vi "OE2052_Configure Channel Out.vi"(7 "OE2052_Configure Channel Out":T1={"Channel Output"=0, "Channel Source"=0, "Offset(%)"=0.0, "Expand"=1, "AUX OUT"=1.0, "Sensitivity "=24} {"Sensitivity" items=["1 nV/fA", "2 nV/fA", "5 nV/fA", "10 nV/fA", "20 nV/fA", "50 nV/fA", "100 nV/fA", "200 nV/fA", "500 nV/fA", "1 uV/pA", "2 uV/pA", "5 uV/pA", "10 uV/pA", "20 uV/pA", "50 uV/pA", "100 uV/pA", "200 uV/pA", "500 uV/pA", "1 mV/nA", "2 mV/nA", "5 mV/nA", "10 mV/nA", "20 mV/nA", "50 mV/nA", "100 mV/nA", "200 mV/nA", "500 mV/nA", "1 V/uA"]; "AUX OUT" min=-10.0 max=10.0 format="%#.3g"; "Expand" min=1 max=10000; "Offset(%)" min=-100.0 max=100.0 format="%#_5g"; "Channel Source" items=["AUXOUT", "X1", "Y1", "R1", "θ1", "X2", "Y2", "R2", "θ2", "Frequency1", "Frequency2", "AUX-IN1", "AUX-IN2", "AUX-IN3", "AUX-IN4", "X3", "Y3", "R3", "Xita3", "X4", "Y4", "R4", "Xita4"]; "Channel Output" items=["CH1", "CH2", "CH3", "CH4"]}, 8 "Error in (no error)":errorcluster caption="error out（no error）", 9 "Remote Mode":u16(ring) items=["USB"=0, "RS232"=1, "Ethernet"=3], 10 "Connection ID in":refnum<k5>, 11 "VISA resource name":refnum<visa-resource-name>) -> (0 "Error out":errorcluster caption="error out", 1 "Output String":string, 2 "Connection ID out":refnum<k5>, 3 "VISA resource  out":refnum<visa-resource-name>)   [LabVIEW 2011]
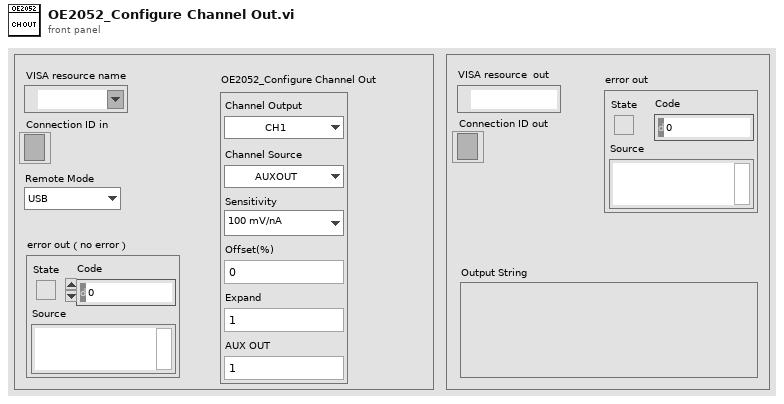
[diagram p1: front panel]
types:
  T1 = cluster{"Channel Output":u16, "Channel Source":u16, "Offset(%)":dbl, "Expand":u16, "AUX OUT":dbl, "Sensitivity ":u16}
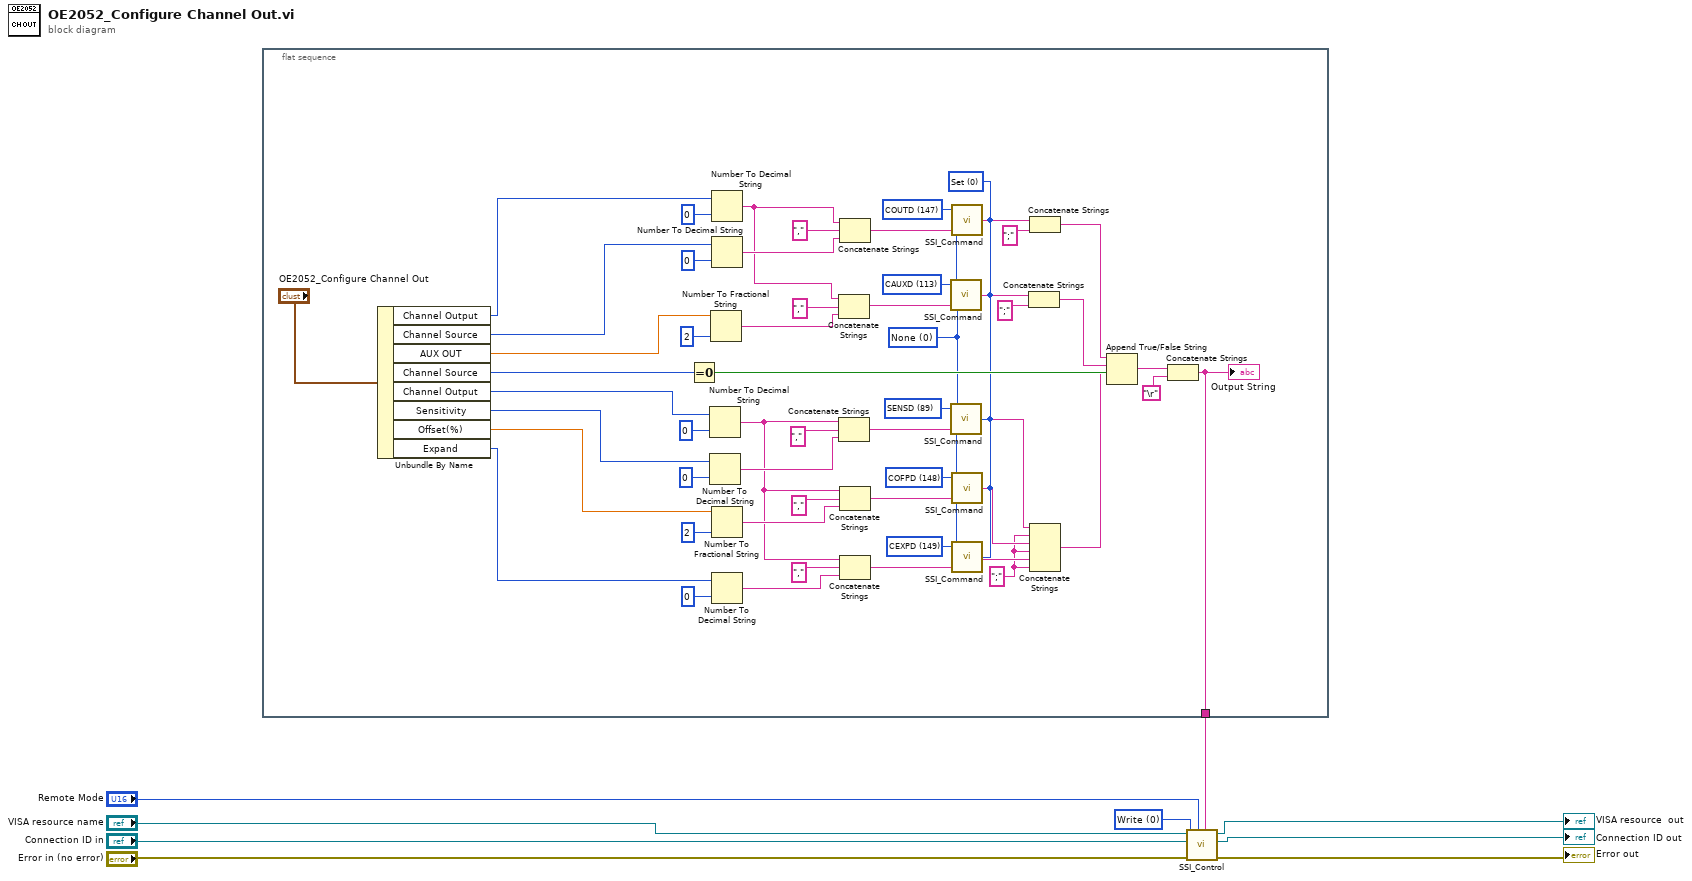
[diagram p0: block diagram]
diagram:
  w2 = u16 0 items=["Write", "Read"] ("Control")
  n1 = flat-sequence {
    tunnel: [w40] -> w1
    frame #0 {
      w11 = u16 0 items=["A"=1, "B"=2, "None"=0] ("channel")
      w20 = u16 149 items=["ISRC", "IGND", "ICPL", "ILIN", "PHAS", "FMOD", "RSLP", "FREQ", "SWPT", "SLLM", "SULM", "SSLL", "SSLG", "STLM", "SWRM", "IRNG", "SENS", "RMOD", "OFLT", "OFSL", "SYNC", "DMOD", "HARM", "DARB", "SWVT", "SLVL", "SVLL", "SVUL", "SVSL", "SVSG", "SVTM", "SVRM", "RALL", "SNAP", "OUTP", "OAUX", "COUT", "CAUX", "COFP", "CEXP", "FPOP", "OEXP", "*IDN", "*RST", "OVLD", "INOV", "GNOV", "*PLL", "SSET", "RSET", "AGAN", "APHS", "ARSV", "ASCL", "EQCD", "EQCS", "SPED", "SRAT", "SLEN", "SSLE", "STRG", "SPRM", "STRD", "PAUS", "REST", "SPTS", "TRCA", "TEMP", "RSTU", "INHZ", "DEQU", "SADD", "ARNG", "CSPE", "ISRCD", "IGNDD", "ICPLD", "ILIND", "PHASD", "FMODD", "RSLPD", "FREQD", "SWPTD", "SLLMD", "SULMD", "SSLLD", "SSLGD", "STLMD", "SWRMD", "SENSD", "RMODD", "OFLTD", "OFSLD", "SYNCD", "HARMD", "EQCDD", "EQCSD", "SNAPD", "OUTPD", "SWVTD", "SLVLD", "SVLLD", "SVULD", "SVSLD", "SVSGD", "SVTMD", "SVRMD", "SVDCD", "ARSVD", "AGAND", "APHSD", "ASCLD", "FPOPD", "CAUXD", "OEXPD", "SPEDD", "SRATD", "SLEND", "SSLED", "STRGD", "SPRMD", "STRDD", "PAUSD", "RESTD", "SPTSD", "TRCAD", "*IDND", "*RSTD", "INOVD", "GNOVD", "*PLLD", "SSETD", "RSETD", "RALLD", "NIPA", "NSMA", "NGWA", "NMAC", "NMOD", "TRIG", "TRCB", "INHZD", "ISAMD", "IRAGD", "RRAGD", "SOFFD", "DMODD", "COUTD", "COFPD", "CEXPD", "ARNGD", "OAUXD", "TRIM", "SUITD", "SNHZD", "AOFSD"] ("Command Type")
      w21 = u16 148 items=["ISRC", "IGND", "ICPL", "ILIN", "PHAS", "FMOD", "RSLP", "FREQ", "SWPT", "SLLM", "SULM", "SSLL", "SSLG", "STLM", "SWRM", "IRNG", "SENS", "RMOD", "OFLT", "OFSL", "SYNC", "DMOD", "HARM", "DARB", "SWVT", "SLVL", "SVLL", "SVUL", "SVSL", "SVSG", "SVTM", "SVRM", "RALL", "SNAP", "OUTP", "OAUX", "COUT", "CAUX", "COFP", "CEXP", "FPOP", "OEXP", "*IDN", "*RST", "OVLD", "INOV", "GNOV", "*PLL", "SSET", "RSET", "AGAN", "APHS", "ARSV", "ASCL", "EQCD", "EQCS", "SPED", "SRAT", "SLEN", "SSLE", "STRG", "SPRM", "STRD", "PAUS", "REST", "SPTS", "TRCA", "TEMP", "RSTU", "INHZ", "DEQU", "SADD", "ARNG", "CSPE", "ISRCD", "IGNDD", "ICPLD", "ILIND", "PHASD", "FMODD", "RSLPD", "FREQD", "SWPTD", "SLLMD", "SULMD", "SSLLD", "SSLGD", "STLMD", "SWRMD", "SENSD", "RMODD", "OFLTD", "OFSLD", "SYNCD", "HARMD", "EQCDD", "EQCSD", "SNAPD", "OUTPD", "SWVTD", "SLVLD", "SVLLD", "SVULD", "SVSLD", "SVSGD", "SVTMD", "SVRMD", "SVDCD", "ARSVD", "AGAND", "APHSD", "ASCLD", "FPOPD", "CAUXD", "OEXPD", "SPEDD", "SRATD", "SLEND", "SSLED", "STRGD", "SPRMD", "STRDD", "PAUSD", "RESTD", "SPTSD", "TRCAD", "*IDND", "*RSTD", "INOVD", "GNOVD", "*PLLD", "SSETD", "RSETD", "RALLD", "NIPA", "NSMA", "NGWA", "NMAC", "NMOD", "TRIG", "TRCB", "INHZD", "ISAMD", "IRAGD", "RRAGD", "SOFFD", "DMODD", "COUTD", "COFPD", "CEXPD", "ARNGD", "OAUXD", "TRIM", "SUITD", "SNHZD", "AOFSD"] ("Command Type")
      w22 = u16 89 items=["ISRC", "IGND", "ICPL", "ILIN", "PHAS", "FMOD", "RSLP", "FREQ", "SWPT", "SLLM", "SULM", "SSLL", "SSLG", "STLM", "SWRM", "IRNG", "SENS", "RMOD", "OFLT", "OFSL", "SYNC", "DMOD", "HARM", "DARB", "SWVT", "SLVL", "SVLL", "SVUL", "SVSL", "SVSG", "SVTM", "SVRM", "RALL", "SNAP", "OUTP", "OAUX", "COUT", "CAUX", "COFP", "CEXP", "FPOP", "OEXP", "*IDN", "*RST", "OVLD", "INOV", "GNOV", "*PLL", "SSET", "RSET", "AGAN", "APHS", "ARSV", "ASCL", "EQCD", "EQCS", "SPED", "SRAT", "SLEN", "SSLE", "STRG", "SPRM", "STRD", "PAUS", "REST", "SPTS", "TRCA", "TEMP", "RSTU", "INHZ", "DEQU", "SADD", "ARNG", "CSPE", "ISRCD", "IGNDD", "ICPLD", "ILIND", "PHASD", "FMODD", "RSLPD", "FREQD", "SWPTD", "SLLMD", "SULMD", "SSLLD", "SSLGD", "STLMD", "SWRMD", "SENSD", "RMODD", "OFLTD", "OFSLD", "SYNCD", "HARMD", "EQCDD", "EQCSD", "SNAPD", "OUTPD", "SWVTD", "SLVLD", "SVLLD", "SVULD", "SVSLD", "SVSGD", "SVTMD", "SVRMD", "SVDCD", "ARSVD", "AGAND", "APHSD", "ASCLD", "FPOPD", "CAUXD", "OEXPD", "SPEDD", "SRATD", "SLEND", "SSLED", "STRGD", "SPRMD", "STRDD", "PAUSD", "RESTD", "SPTSD", "TRCAD", "*IDND", "*RSTD", "INOVD", "GNOVD", "*PLLD", "SSETD", "RSETD", "RALLD", "NIPA", "NSMA", "NGWA", "NMAC", "NMOD", "TRIG", "TRCB", "INHZD", "ISAMD", "IRAGD", "RRAGD", "SOFFD", "DMODD", "COUTD", "COFPD", "CEXPD", "ARNGD", "OAUXD", "TRIM", "SUITD", "SNHZD", "AOFSD"] ("Command Type")
      w30 = u16 113 items=["ISRC", "IGND", "ICPL", "ILIN", "PHAS", "FMOD", "RSLP", "FREQ", "SWPT", "SLLM", "SULM", "SSLL", "SSLG", "STLM", "SWRM", "IRNG", "SENS", "RMOD", "OFLT", "OFSL", "SYNC", "DMOD", "HARM", "DARB", "SWVT", "SLVL", "SVLL", "SVUL", "SVSL", "SVSG", "SVTM", "SVRM", "RALL", "SNAP", "OUTP", "OAUX", "COUT", "CAUX", "COFP", "CEXP", "FPOP", "OEXP", "*IDN", "*RST", "OVLD", "INOV", "GNOV", "*PLL", "SSET", "RSET", "AGAN", "APHS", "ARSV", "ASCL", "EQCD", "EQCS", "SPED", "SRAT", "SLEN", "SSLE", "STRG", "SPRM", "STRD", "PAUS", "REST", "SPTS", "TRCA", "TEMP", "RSTU", "INHZ", "DEQU", "SADD", "ARNG", "CSPE", "ISRCD", "IGNDD", "ICPLD", "ILIND", "PHASD", "FMODD", "RSLPD", "FREQD", "SWPTD", "SLLMD", "SULMD", "SSLLD", "SSLGD", "STLMD", "SWRMD", "SENSD", "RMODD", "OFLTD", "OFSLD", "SYNCD", "HARMD", "EQCDD", "EQCSD", "SNAPD", "OUTPD", "SWVTD", "SLVLD", "SVLLD", "SVULD", "SVSLD", "SVSGD", "SVTMD", "SVRMD", "SVDCD", "ARSVD", "AGAND", "APHSD", "ASCLD", "FPOPD", "CAUXD", "OEXPD", "SPEDD", "SRATD", "SLEND", "SSLED", "STRGD", "SPRMD", "STRDD", "PAUSD", "RESTD", "SPTSD", "TRCAD", "*IDND", "*RSTD", "INOVD", "GNOVD", "*PLLD", "SSETD", "RSETD", "RALLD", "NIPA", "NSMA", "NGWA", "NMAC", "NMOD", "TRIG", "TRCB", "INHZD", "ISAMD", "IRAGD", "RRAGD", "SOFFD", "DMODD", "COUTD", "COFPD", "CEXPD", "ARNGD", "OAUXD", "TRIM", "SUITD", "SNHZD", "AOFSD"] ("Command Type")
      w34 = u16 147 items=["ISRC", "IGND", "ICPL", "ILIN", "PHAS", "FMOD", "RSLP", "FREQ", "SWPT", "SLLM", "SULM", "SSLL", "SSLG", "STLM", "SWRM", "IRNG", "SENS", "RMOD", "OFLT", "OFSL", "SYNC", "DMOD", "HARM", "DARB", "SWVT", "SLVL", "SVLL", "SVUL", "SVSL", "SVSG", "SVTM", "SVRM", "RALL", "SNAP", "OUTP", "OAUX", "COUT", "CAUX", "COFP", "CEXP", "FPOP", "OEXP", "*IDN", "*RST", "OVLD", "INOV", "GNOV", "*PLL", "SSET", "RSET", "AGAN", "APHS", "ARSV", "ASCL", "EQCD", "EQCS", "SPED", "SRAT", "SLEN", "SSLE", "STRG", "SPRM", "STRD", "PAUS", "REST", "SPTS", "TRCA", "TEMP", "RSTU", "INHZ", "DEQU", "SADD", "ARNG", "CSPE", "ISRCD", "IGNDD", "ICPLD", "ILIND", "PHASD", "FMODD", "RSLPD", "FREQD", "SWPTD", "SLLMD", "SULMD", "SSLLD", "SSLGD", "STLMD", "SWRMD", "SENSD", "RMODD", "OFLTD", "OFSLD", "SYNCD", "HARMD", "EQCDD", "EQCSD", "SNAPD", "OUTPD", "SWVTD", "SLVLD", "SVLLD", "SVULD", "SVSLD", "SVSGD", "SVTMD", "SVRMD", "SVDCD", "ARSVD", "AGAND", "APHSD", "ASCLD", "FPOPD", "CAUXD", "OEXPD", "SPEDD", "SRATD", "SLEND", "SSLED", "STRGD", "SPRMD", "STRDD", "PAUSD", "RESTD", "SPTSD", "TRCAD", "*IDND", "*RSTD", "INOVD", "GNOVD", "*PLLD", "SSETD", "RSETD", "RALLD", "NIPA", "NSMA", "NGWA", "NMAC", "NMOD", "TRIG", "TRCB", "INHZD", "ISAMD", "IRAGD", "RRAGD", "SOFFD", "DMODD", "COUTD", "COFPD", "CEXPD", "ARNGD", "OAUXD", "TRIM", "SUITD", "SNHZD", "AOFSD"] ("Command Type")
      w12 = ";" ("字符串")
      w27 = u16 0 items=["Set", "Query"] ("Opera")
      n2 = Unbundle By Name("OE2052_Configure Channel Out") -> ("Channel Output"=w33:u16, "Channel Source"=w31:u16, "AUX OUT"=w32:dbl, "Channel Source"=w10:u16, "Channel Output"=w17:u16, "Sensitivity"=w25:u16, "Offset(%)"=w15:dbl, "Expand"=w14:u16)
      n3 = Equal To 0?(x=w10) -> (x = 0?=w52:bool)
      n4 = Number To Decimal String(number=w17, width (-)=i16 0 ("精度(6)")) -> (decimal integer string=w16:string)
      n5 = Number To Decimal String(number=w25, width (-)=i16 0 ("精度(6)")) -> (decimal integer string=w24:string)
      n6 = Number To Fractional String(number=w32, precision (6)=i16 2 ("精度(6)")) -> (F-format string=w38:string)  [unwired: 2 in]
      n7 = Number To Decimal String(number=w33, width (-)=i16 0 ("精度(6)")) -> (decimal integer string=w19:string)
      n8 = Number To Decimal String(number=w31, width (-)=i16 0 ("精度(6)")) -> (decimal integer string=w54:string)
      n9 = Number To Fractional String(number=w15, precision (6)=i16 2 ("精度(6)")) -> (F-format string=w48:string)  [unwired: 2 in]
      n10 = Number To Decimal String(number=w14, width (-)=i16 0 ("精度(6)")) -> (decimal integer string=w13:string)
      n11 = Concatenate Strings(w19, "," ("字符串"), w38) -> (w37:string)
      n12 = Concatenate Strings(w16, "," ("字符串"), w24) -> (w29:string)
      n13 = Concatenate Strings(w19, "," ("字符串"), w54) -> (w55:string)
      n14 = Concatenate Strings(w16, "," ("字符串"), w48) -> (w49:string)
      n15 = Concatenate Strings(w16, "," ("字符串"), w13) -> (w46:string)
      n16 = call "SSI_Command.vi"("Opera"=w27, "Paramter"=w37, "channel"=w11, "Command Type"=w30) -> ("Output string"=w63:string)
      n17 = call "SSI_Command.vi"("Opera"=w27, "Paramter"=w29, "channel"=w11, "Command Type"=w22) -> ("Output string"=w23:string)
      n18 = call "SSI_Command.vi"("Opera"=w27, "Paramter"=w55, "channel"=w11, "Command Type"=w34) -> ("Output string"=w61:string)
      n19 = call "SSI_Command.vi"("Opera"=w27, "Paramter"=w49, "channel"=w11, "Command Type"=w21) -> ("Output string"=w44:string)
      n20 = call "SSI_Command.vi"("Opera"=w27, "Paramter"=w46, "channel"=w11, "Command Type"=w20) -> ("Output string"=w60:string)
      n21 = Concatenate Strings(w63, ";" ("替换字符串(\"\")")) -> (w51:string)
      n22 = Concatenate Strings(w61, ";" ("替换字符串(\"\")")) -> (w35:string)
      n23 = Concatenate Strings(w23, w12, w44, w12, w60, w12) -> (w41:string)
      n24 = Append True/False String(1:w52, 2:w41, 3:w51, 4:w35) -> (0:w42:string)
      n25 = Concatenate Strings(w42, "\r") -> (w40:string)
      "Output String" <- w40
    }
  }
  n26 = call "SSI_Control.vi"("Write Buffer"=w1, "Remote Mode"="Remote Mode", "Error in (no error)"="Error in (no error)", "Control"=w2, "Connection ID in"="Connection ID in", "VISA resource name"="VISA resource name") -> ("Error out"=→"Error out":errorcluster, "Connection ID out"=→"Connection ID out":refnum<k5>, "VISA resource  out"=→"VISA resource  out":refnum<visa-resource-name>)  [unwired: 2 in, 1 out]
